vi "GenerateMethodURL.vi"(7 "Method":enum16{"Heartbeat", "GetSRs"}(ring), 11 "TestClientData":T1) -> (3 "String":string)   [LabVIEW 2017, in "Server.lvlib" / "Dialogs.lvlib"]
uses:
  Dialogs.lvlib
  TestClientData.ctl
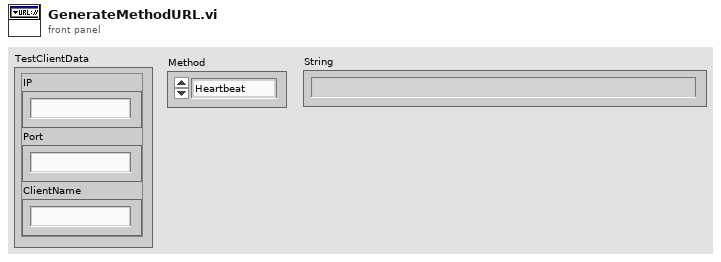
[diagram p1: front panel]
types:
  T1 = typedef "Server.lvlib/Dialogs.lvlib/TestClientData.ctl" = cluster{"IP":string, "Port":string, "ClientName":string}
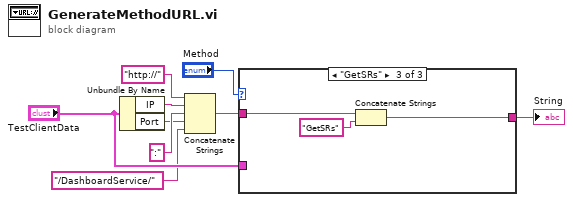
[diagram p0: block diagram]
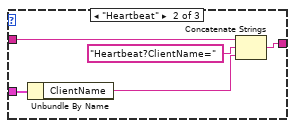
[diagram p3: hidden frame]
diagram:
  n1 = Unbundle By Name("TestClientData") -> ("IP"=w5:string, "Port"=w3:string)
  n2 = Concatenate Strings("http://" ("string"), w5, ":" ("string"), w3, "/DashboardService/" ("string")) -> (w1:string)
  n3 = case shown="\"GetSRs\"" "Method" {
    tunnel: [_ w13 w15] -> w9
    tunnel: "TestClientData" -> [_ w12 _]
    tunnel: w1 -> [_ w10 w17]
    frame Default {
    }
    frame "Heartbeat" {
      n4 = Unbundle By Name(w12) -> ("ClientName"=w11:string)
      n5 = Concatenate Strings(w10, "Heartbeat?ClientName=" ("string"), w11) -> (w13:string)
    }
    frame "GetSRs" {
      n6 = Concatenate Strings(w17, "GetSRs" ("string")) -> (w15:string)
    }
  }
  "String" <- w9
